vi "Drive Controller.vi"(8 "error in":errorcluster) -> ()   [LabVIEW 2019]
doc: "This VI executes continuously carrying out the current operation and responding to updates or new operation requests. It will often contain the timing or control code that is difficult to place directly in TeleOp. This VI generally opens all sensors and motors and isolates the rest of the robot code from knowing implementation details of how the operations are carried out."
uses:
  <vilib>/Rock Robotics/WPI/Framework/Completion Status.ctl
  Drive Setpoints.ctl
  Drive Operations.ctl
  <vilib>/Rock Robotics/WPI/ThirdParty/REV Robotics/SPARK MAX/Typedef/Spark MAX Control Type.ctl
  Odometry/ADIS16470/Typedef/ADIS16470 Hardware Configuration.ctl
  <vilib>/Rock Robotics/WPI/SPI/WPI_SPIMode.ctl
  <vilib>/Rock Robotics/SystemInterfaces/DIO/FPGA_DIOChannel.ctl
  <vilib>/Rock Robotics/SystemInterfaces/spilib/spi_bus.ctl
  <vilib>/Rock Robotics/WPI/ThirdParty/WPILib Extensions/Geometry/Typedef/Pose2d.ctl
  <vilib>/Rock Robotics/WPI/ThirdParty/WPILib Extensions/Geometry/Typedef/Translation2d.ctl
  <vilib>/Rock Robotics/WPI/ThirdParty/WPILib Extensions/Geometry/Typedef/Rotation2d.ctl
  <vilib>/Rock Robotics/WPI/Gyro/WPI_GyroDevRef.ctl
  <vilib>/Rock Robotics/SystemInterfaces/AI/FPGA_AIChannel.ctl
  CAN Functions/SPARKMAX6Motor.ctl
  <vilib>/Rock Robotics/WPI/MotorControl/WPI_MotorControlDeviceRef.ctl
  <vilib>/Rock Robotics/WPI/MotorControl/WPI_MotorControlType.ctl
  <vilib>/Rock Robotics/SystemInterfaces/DIO/FPGA_DIOPWMChannel.ctl
  <vilib>/Rock Robotics/WPI/PWM/WPI_PWMDeadband.ctl
  <vilib>/Rock Robotics/WPI/ThirdParty/WPILib Extensions/Controller/PID/Typedef/PID Controller State.ctl
  Odometry/ADIS16470/Typedef/ADIS16470 Calibration Time.ctl
  Odometry/Typedef/Odometry.ctl
  Odometry/Typedef/Velocity Data.ctl
  Pure Pursuit/Typedef/Pure Pursuit Telemetry.ctl
  Pure Pursuit/Typedef/Path Point.ctl
  <vilib>/Rock Robotics/WPI/ThirdParty/WPILib Extensions/Trajectory/Typedef/Trajectory State.ctl
  <vilib>/Rock Robotics/WPI/Counter/WPI_CounterDigitalInputToDigitalSource.vi
  Odometry/Odometry Set.vi
  <vilib>/ptbypt/NI_PtbyPt.lvlib
  Pure Pursuit/Pure Pursuit.lvlib
panel:
  in  "Drive Distance Tolerance":dbl format="%#_13g"
  in  "ADIS16470 Config":T1={"SPI Clock Rate (Hz)"=2000000.0, "IMU SPI Mode (3)"=enum."Mode 3 (Clk Idle High,Sample on Trailing)", "IMU Reset Pin"=enum."SPI Port CS2", "IMU SPI Bus"=enum."SPI On-Board, CS0", "IMU Data Ready Pin"=enum."SPI Port CS1", "Stall Config"={"Pow2BytesPerRead"=1, "StallTicks"=1000, "CsToSclkTicks"=5}}
  in  "Trackwidth":dbl=0.6716296994500001
  in  "Control Mode":T5
  in  "Tab Control":T6(tab)=enum."Settings"
  in  "Interactive Values":T7
  in  "Buttons":cluster{"Execute Cmd":bool, "Abort Cmd":bool}
  out "Command Timing":cluster{"Start Time (ms)":u32, "Iterations":i32}={"Start Time (ms)"=2524017, "Iterations"=0}
  out "Status":T9
  in  "PID Constants Drivetrain":T10={"P Gain"=1.0, "I Gain"=0.0, "D Gain"=0.0, "F Gain"=0.0, "I Zone"=0.0, "Min Output"=-1.0, "Max Output"=1.0} {"Max Output" min=-1.0 max=1.0 step=0.01; "Min Output" min=-1.0 max=1.0 step=0.01; "I Zone" step=0.01; "F Gain" step=0.01; "D Gain" step=0.01; "I Gain" step=0.01; "P Gain" min=0.0 step=0.01}
  in  "Trackwidth":dbl=0.6716296994500001 format="%#_13g"
  in  "Max Velocity":dbl=2.0
  in  "Max Accel":dbl=4.0
  in  "Lookahead":dbl=18.0
  in  "kffv":dbl
  in  "kffa":dbl=0.05
  in  "Feed Forward":cluster{"kS":dbl, "kV":dbl, "kA":dbl}={"kS"=0.162, "kV"=2.71, "kA"=0.468}
  in  "Encoder Factor":dbl=0.00030795
  out "Pose":T11
  in  "Value":dbl
  in  "Run":bool
  out "Waveform Chart":dbl(graph)
  out "XY Graph":cluster{"X":dbl, "Y":dbl}[](graph)
  in  "Test":string(combo)="quasi-static ramp"
  out "Telemetry":cluster{dbl[], dbl[]}[](graph)
  in  "Output Range":cluster{"output high":dbl, "output low":dbl}
  in  "Profiled Contraints":T14
  in  "PIDF Gains":cluster{"Kp":dbl, "Ki":dbl, "Kd":dbl, "Kf":dbl}
  in  "Gyro PIDF":cluster{"Kp":dbl, "Ki":dbl, "Kd":dbl, "Kf":dbl}={"Kp"=0.05, "Ki"=0.0, "Kd"=0.0, "Kf"=0.0} {"Kf" format="%.3f"; "Kd" format="%.3f"; "Ki" format="%.3f"; "Kp" format="%.3f"}
  out "Current\nCmd":string="Started at  20:49:40.426\nDefault: Reserve,  L 0.0, R 0.0, D 0.000000"
  # "Click here to set min"
  # "Interactive Command: You may fill in the settings for a command\nand schedule it with the Execute button. You can observe and abort\nany command while fine tuning the code for the controller."
  # "Pure Pursuit"
  # "Velocity Control is the Output (m/s)"
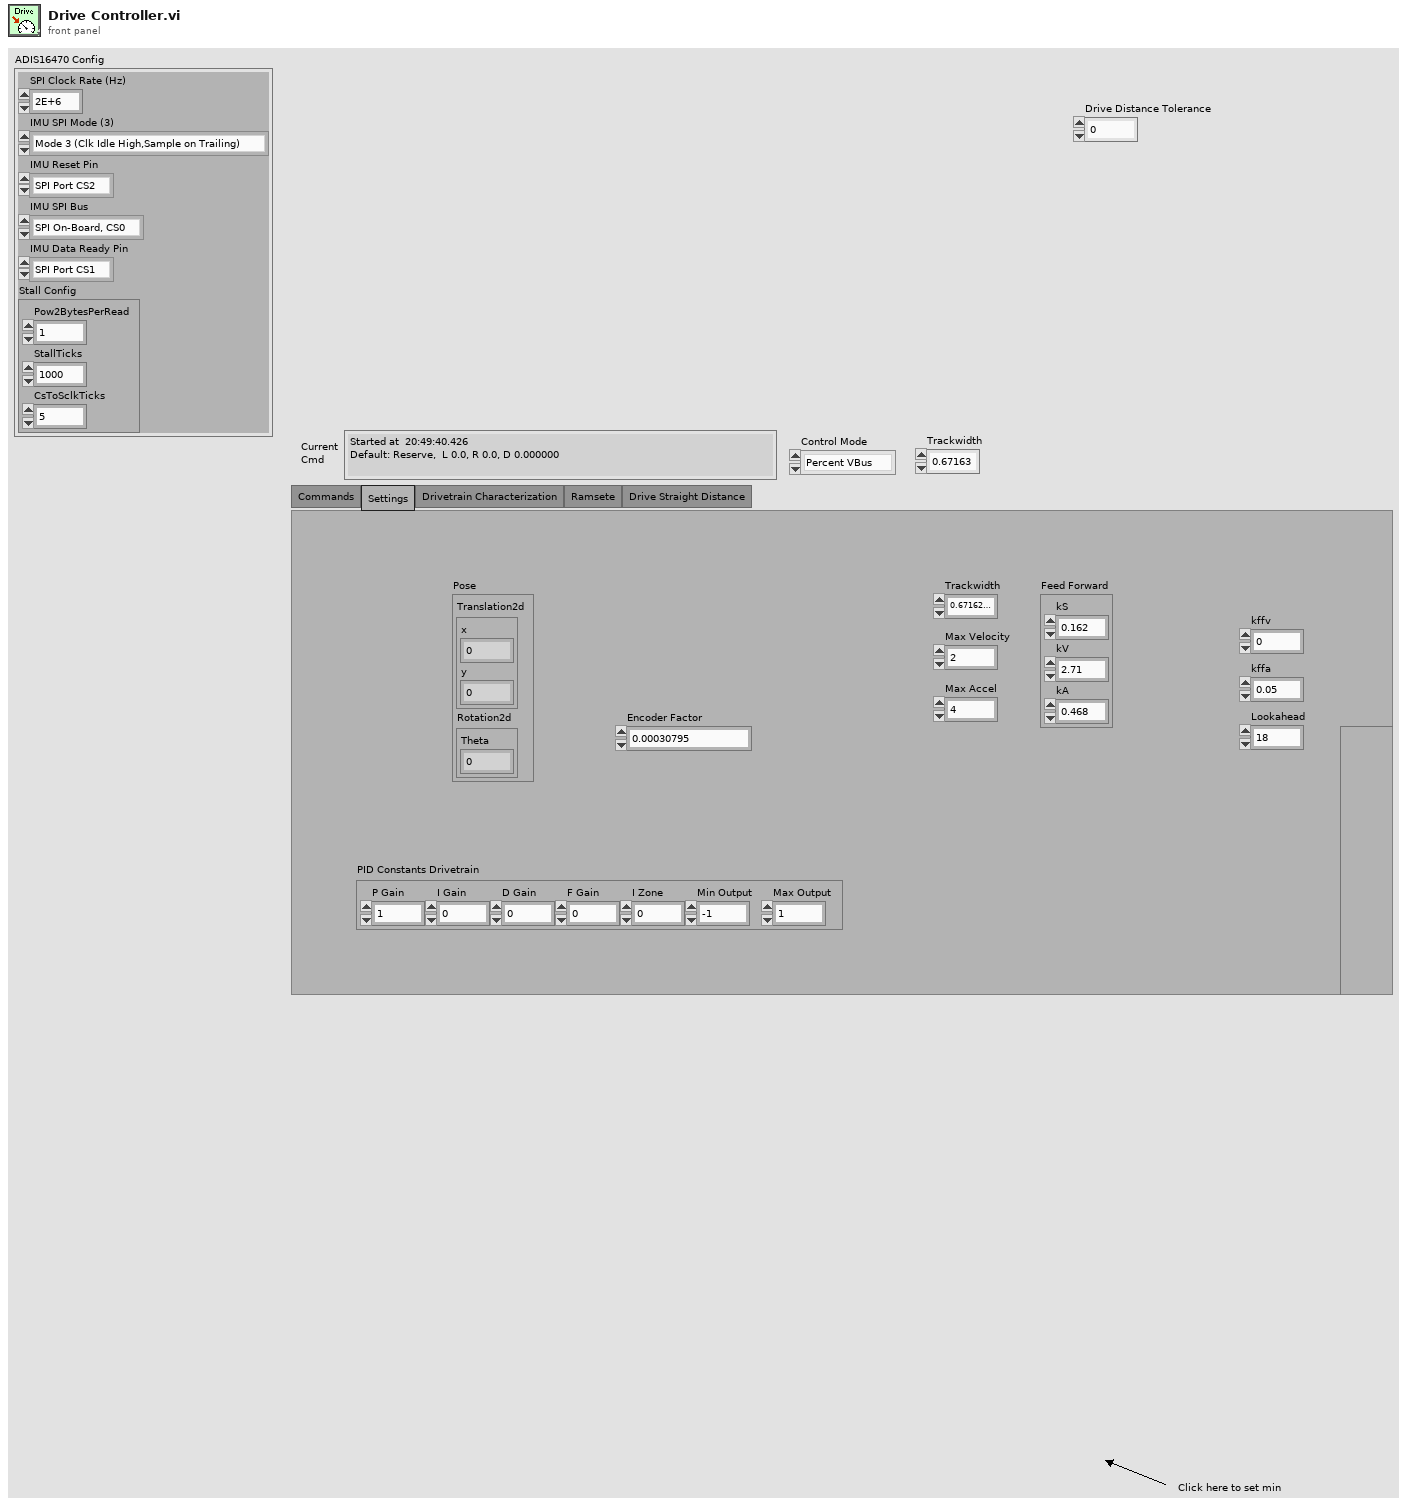
[diagram p1: front panel]
types:
  T1 = typedef "ADIS16470 Hardware Configuration.ctl" = cluster{"SPI Clock Rate (Hz)":dbl, "IMU SPI Mode (3)":T2, "IMU Reset Pin":T3, "IMU SPI Bus":T4, "IMU Data Ready Pin":T3, "Stall Config":cluster{"Pow2BytesPerRead":u8, "StallTicks":u16, "CsToSclkTicks":u8}}
  T2 = typedef "WPI_SPIMode.ctl" = enum16{"Mode 0 (Clk Idle Low,Sample on Leading)", "Mode 1 (Clk Idle Low,Sample on Trailing)", "Mode 2 (Clk Idle High,Sample on Leading)", "Mode 3 (Clk Idle High,Sample on Trailing)"}
  T3 = typedef "FPGA_DIOChannel.ctl" = enum8{"DIO 0", "DIO 1", "DIO 2", "DIO 3", "DIO 4", "DIO 5", "DIO 6", "DIO 7", "DIO 8", "DIO 9", "DIO MXP 0", "DIO MXP 1", "DIO MXP 2", "DIO MXP 3", "DIO MXP 4", "DIO MXP 5", "DIO MXP 6", "DIO MXP 7", "DIO MXP 8", "DIO MXP 9", "DIO MXP 10", "DIO MXP 11", "DIO MXP 12", "DIO MXP 13", "DIO MXP 14", "DIO MXP 15", "SPI Port CS1", "SPI Port CS2", "SPI Port CS3", "SPI Port MISO", "SPI Port MOSI", "Invalid"}
  T4 = typedef "spi_bus.ctl" = enum16{"SPI On-Board, CS0", "SPI On-Board, CS1", "SPI On-Board, CS2", "SPI On-Board, CS3", "SPI MXP", "Invalid"}
  T5 = typedef "Spark MAX Control Type.ctl" = enum16{"Percent VBus", "Voltage", "Velocity", "Position", "Smart Motion", "Current", "Smart Velocity"}
  T6 = enum32{"Commands", "Settings", "Drivetrain Characterization", "Ramsete", "Drive Straight Distance"}
  T7 = typedef "Drive Setpoints.ctl" = cluster{"Operation":T8, "Left Setpoint":dbl, "Right Setpoint":dbl, "Duration":dbl, "Data":variant}
  T8 = typedef "Drive Operations.ctl" = enum16{"Reserve", "Read Current", "Immediate", "Drive for Time", "Drive for Distance", "Turn to Angle", "Drivetrain Char", "Pure Pursuit", "Ramsete"}
  T9 = typedef "Completion Status.ctl" = enum16{"Successful", "Aborted", "Incomplete"}
  T10 = cluster{"P Gain":dbl, "I Gain":dbl, "D Gain":dbl, "F Gain":dbl, "I Zone":dbl, "Min Output":dbl, "Max Output":dbl}
  T11 = typedef "Pose2d.ctl" = cluster{"Translation2d":T12, "Rotation2d":T13}
  T12 = typedef "Translation2d.ctl" = cluster{"x":dbl, "y":dbl}
  T13 = typedef "Rotation2d.ctl" = cluster{"Theta":dbl}
  T14 = cluster{"Max Velocity":dbl, "Max Acceleration":dbl}
  T15 = typedef "WPI_GyroDevRef.ctl" = cluster{"DevStatus":errorcluster, "Analog Channel":T16, "Gain (VoltsPerDegree/Second)":dbl, "Gyro Type":enum16{"Analog", "XRS450"}, "Handle":i32, "SPI Bus":T4, "Device Found":bool, "Sample Rate":dbl, "Calibrate On Open":bool, "Offset":dbl}
  T16 = typedef "FPGA_AIChannel.ctl" = enum8{"AI 0", "AI 1", "AI 2", "AI 3", "AI MXP 0", "AI MXP 1", "AI MXP 2", "AI MXP 3", "Invalid"}
  T17 = typedef "SPARKMAX6Motor.ctl" = cluster{"FrontLeftMaster":T18, "FrontLeftSlave1":T18, "FrontLeftSlave2":T18, "FrontRightMaster":T18, "FrontRightSlave1":T18, "FrontRightSlave2":T18}
  T18 = typedef "WPI_MotorControlDeviceRef.ctl" = cluster{"DeviceStatus":errorcluster, "Type":T19, "PWM":cluster{"PWM Channel":T20, "DeadBand":T21}, "CAN":cluster{"Device Number":u8, "SetOutput VI Ref":variant, "GetOutput VI Ref":variant, "Enable VI Ref":variant, "Disable VI Ref":variant, "Data":variant}, "Invert":bool, "DIO PWM":cluster{"PWM \"Enable\" Channel":T20, "DIOChannel":T3, "PWM Rate":dbl}}
  T19 = typedef "WPI_MotorControlType.ctl" = enum16{"PWM", "CAN", "DIO PWM"}
  T20 = typedef "FPGA_DIOPWMChannel.ctl" = enum8{"PWM 0", "PWM 1", "PWM 2", "PWM 3", "PWM 4", "PWM 5", "PWM 6", "PWM 7", "PWM 8", "PWM 9", "PWM MXP 0", "PWM MXP 1", "PWM MXP 2", "PWM MXP 3", "PWM MXP 4", "PWM MXP 5", "PWM MXP 6", "PWM MXP 7", "PWM MXP 8", "PWM MXP 9", "Invalid"}
  T21 = typedef "WPI_PWMDeadband.ctl" = cluster{"Name":string, "maxPositivePwm":i32, "minPositivePwm":i32, "centerPwm":i32, "maxNegativePwm":i32, "minNegativePwm":i32, "angularRange":u16}
  T22 = cluster{"Gyro":T15, "Drivetrain":T17, "PID Ref":refnum<data-value>}
  T23 = typedef "ADIS16470 Calibration Time.ctl" = enum16{"32ms", "64ms", "128ms", "256ms", "512ms", "1s", "2s", "4s", "8s", "16s", "32s", "64s"}
  T24 = typedef "WPI_DigitalInputDevRef.ctl" = cluster{"DevStatus":errorcluster, "DIO Channel":T3}
  T25 = typedef "FPGA_CounterEncoderSourceConvertionLVSourceType.ctl" = cluster{"DevStatus":errorcluster, "AnalogTriggerMode?":bool, "DigitalMode":cluster{"DIO Channel":T26}, "AnalogTriggerMode":cluster{"AnalogTriggerIndex":T27, "OutputType":T28}}
  T26 = typedef "FPGA_DIODigitalSourceChannel.ctl" = enum8{"DIO 0", "DIO 1", "DIO 2", "DIO 3", "DIO 4", "DIO 5", "DIO 6", "DIO 7", "DIO 8", "DIO 9", "DIO MXP 0", "DIO MXP 1", "DIO MXP 2", "DIO MXP 3", "DIO MXP 4", "DIO MXP 5", "DIO MXP 6", "DIO MXP 7", "DIO MXP 8", "DIO MXP 9", "DIO MXP 10", "DIO MXP 11", "DIO MXP 12", "DIO MXP 13", "DIO MXP 14", "DIO MXP 15", "SPI Port CS1", "SPI Port CS2", "SPI Port CS3", "SPI Port MISO", "SPI Port MOSI", "Disabled"}
  T27 = typedef "FPGA_AnalogTriggerIndex.ctl" = enum8{"Trig 0", "Trig 1", "Trig 2", "Trig 3", "Trig 4", "Trig 5", "Trig 6", "Trig 7", "Invalid"}
  T28 = typedef "FPGA_AnalogTriggerOutType.ctl" = enum16{"InWindow", "TriggerState", "Rising", "Falling"}
  T29 = typedef "WPI_EncoderDevRef.ctl" = cluster{"DevStatus":errorcluster, "EncoderIndex":T30, "CounterIndex":T31, "DistancePerCount":dbl, "Decoding Type":T32}
  T30 = typedef "FPGA_EncoderIdx.ctl" = enum8{"Enc 0", "Enc 1", "Enc 2", "Enc 3", "Enc 4", "Enc 5", "Enc 6", "Enc 7", "Invalid"}
  T31 = typedef "FPGA_CounterCtrSystemIndex.ctl" = enum8{"Ctr 0", "Ctr 1", "Ctr 2", "Ctr 3", "Ctr 4", "Ctr 5", "Ctr 6", "Ctr 7", "Invalid"}
  T32 = typedef "WPI_EncoderType.ctl" = enum16{"1x", "2x", "4x"}
  T33 = typedef "ADIS16470 Device Reference.ctl" = cluster{"DevStatus":errorcluster, "Hardware Config":T1, "Calibration Complete":refnum<notifier>, "Status FIFO":refnum<k33>, "Last Value Reference":refnum<data-value>, "Sychronous Process VI":T34, "Cmd FIFO":refnum<k33>, "Source":T25, "Data FIFO":refnum<k33>, "Calibration Time":T23}
  T34 = typedef "ADIS16470 Process.ctl" = refnum<vi>
  T35 = typedef "Command Status Info.ctl" = cluster{"Name":string, "Status":T9, "notifier out":T36}
  T36 = typedef "Completion Notifier.ctl" = refnum<notifier>
  T37 = cluster{"SubSystem Data":T7, cluster{"Start Time (ms)":u32, "Iterations":i32}, cluster{"Command Info":T35, "Description":string, "Default Command":T7, "queue out":refnum<queue>, "Subsystem Name":string}}
  T38 = typedef "Pure Pursuit.lvlib/Pure Pursuit Telemetry.ctl" = cluster{"Target Point":T39, "Close Point":T39, "Curvature":dbl, "index out":i32}
  T39 = typedef "Pure Pursuit.lvlib/Path Point.ctl" = cluster{"x":dbl, "y":dbl, "heading":dbl, "curvature":dbl, "total distance":dbl, "velocity expected":dbl}
  T40 = typedef "Trajectory State.ctl" = cluster{"t":dbl, "velocity":dbl, "acceleration":dbl, "pose":T11, "curvature":dbl}
  T41 = typedef "Odometry.ctl" = cluster{"Left Encoder":dbl, "Right Encoder":dbl, "Late Iterations":u32, "Pose2d":T11}
  T42 = typedef "Velocity Data.ctl" = cluster{"Right Velocity Raw":sgl, "Left Velocity Raw":sgl, "Left Setpoint":dbl, "Right Setpoint":dbl}
  T43 = cluster{"SubSystem Data":T7, cluster{"Start Time (ms)":u32, "Iterations":i32}, "Default Command Arguments":cluster{"Command Info":T35, "Description":string, "Default Command":T7, "queue out":refnum<queue>, "Subsystem Name":string}}
  T44 = cluster{"P Gain":bool, "I Gain":bool, "D Gain":bool, "F Gain":bool, "I Zone":bool, "Min Output":bool, "Max Output":bool}
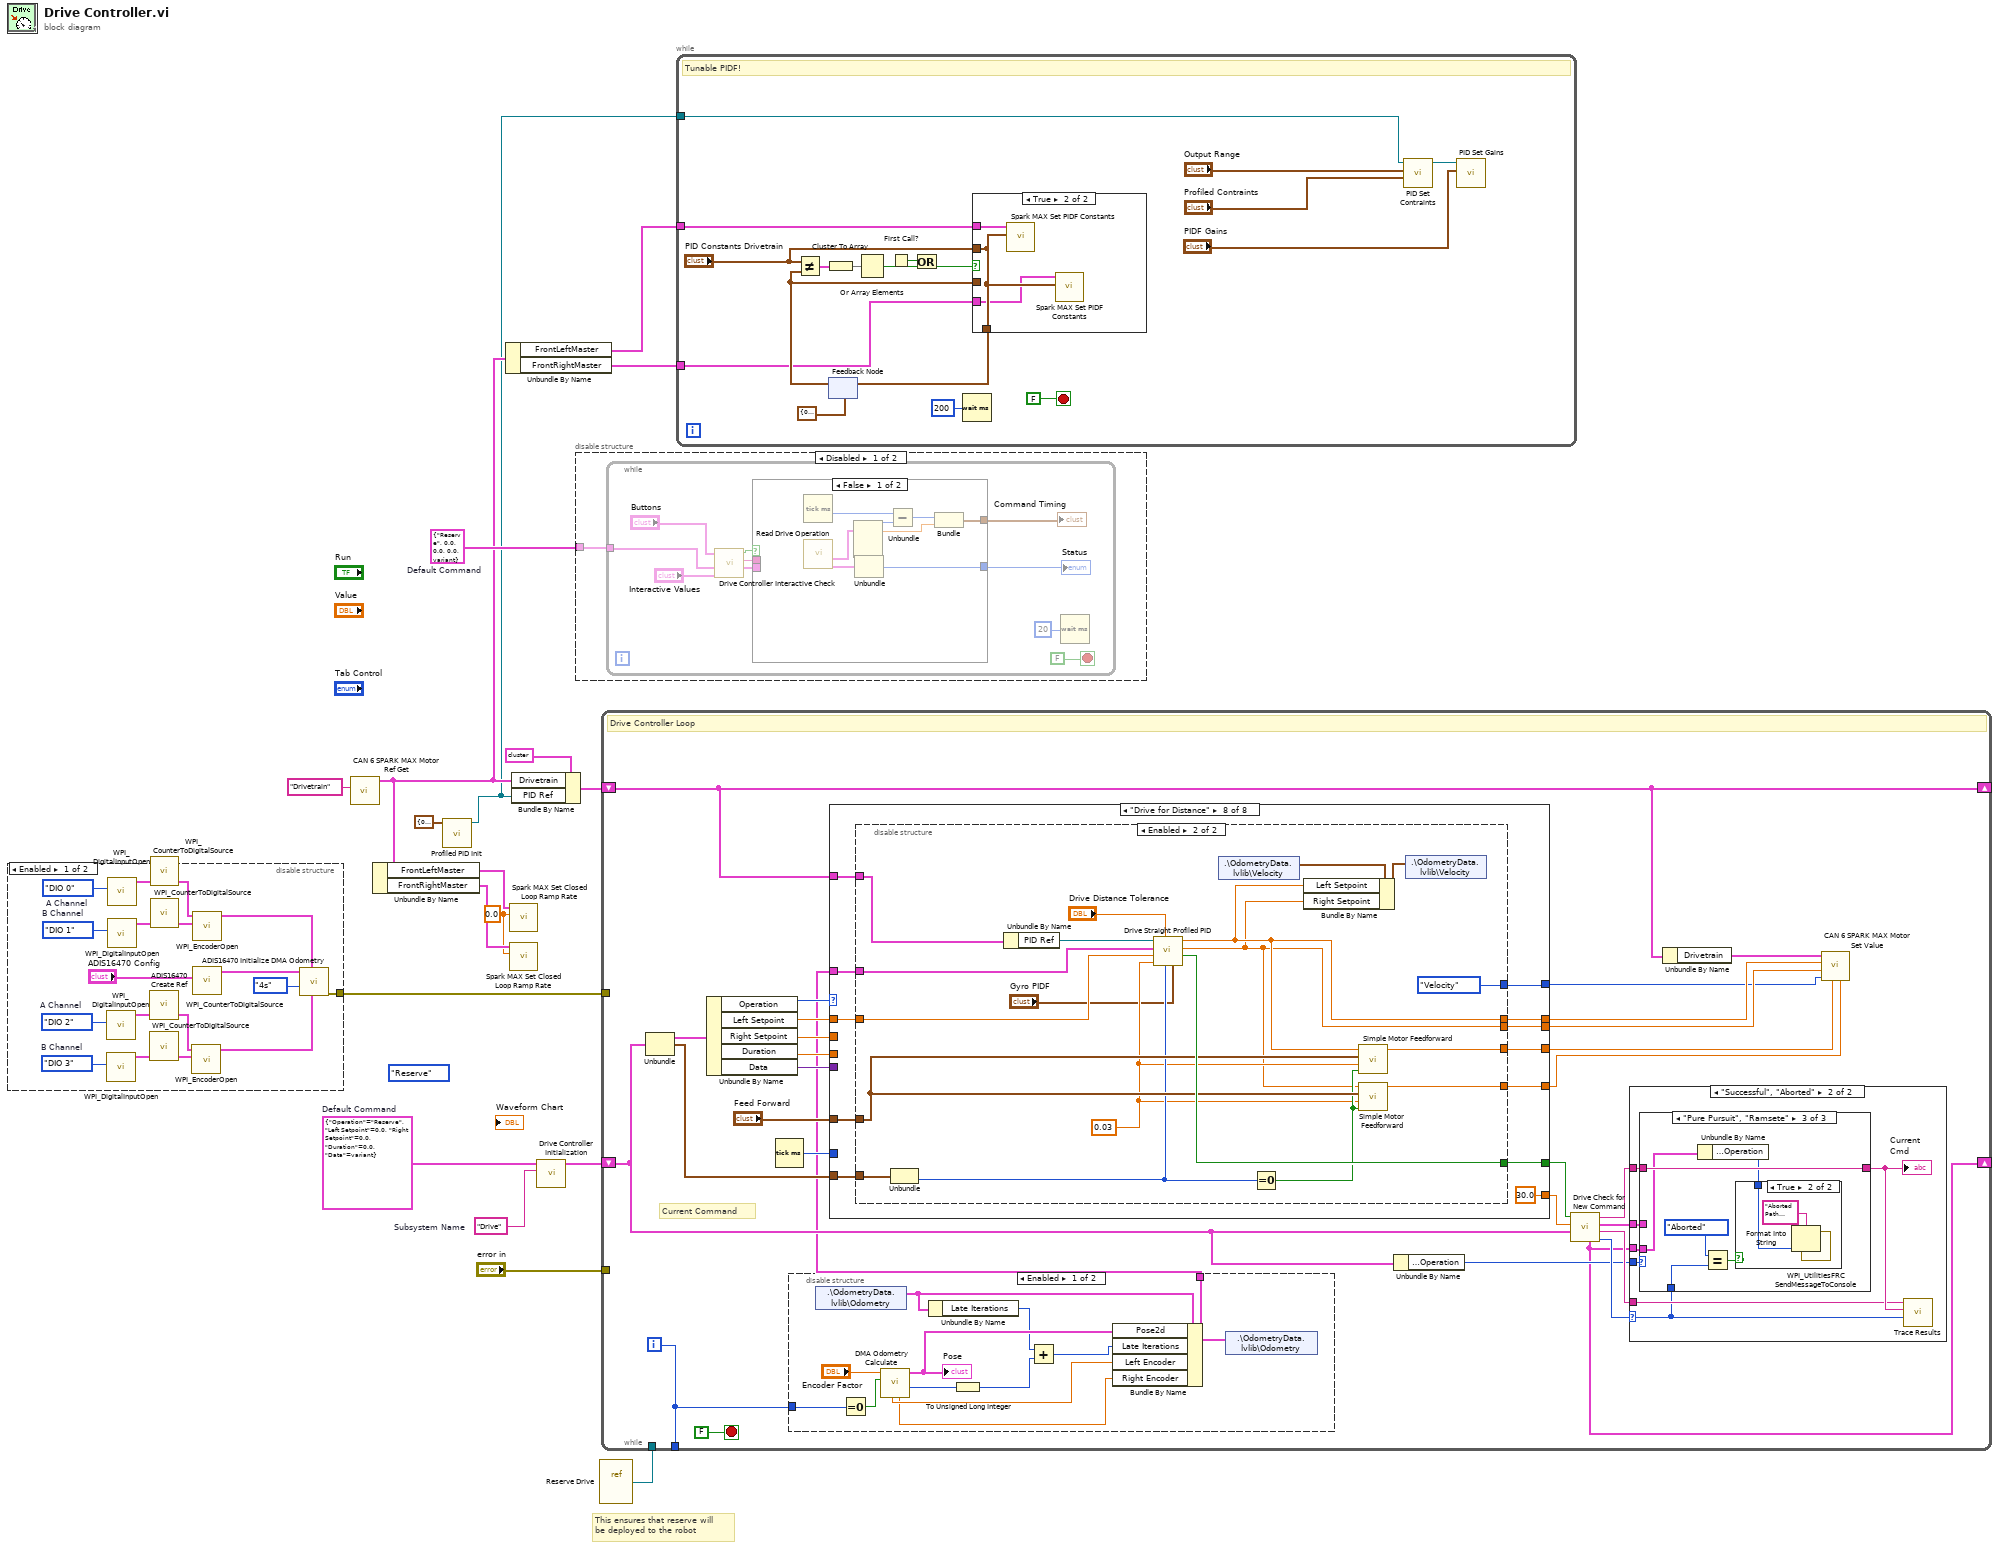
[diagram p0: block diagram]
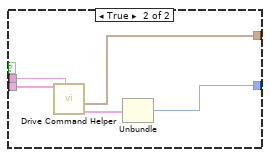
[diagram p3: hidden frame]
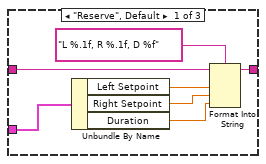
[diagram p7: hidden frame]
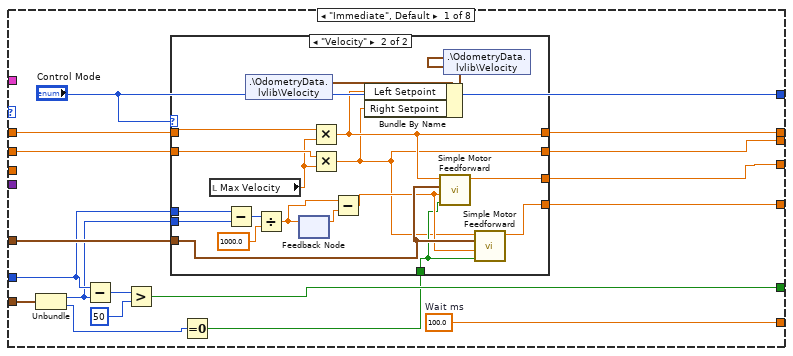
[diagram p10: hidden frame]
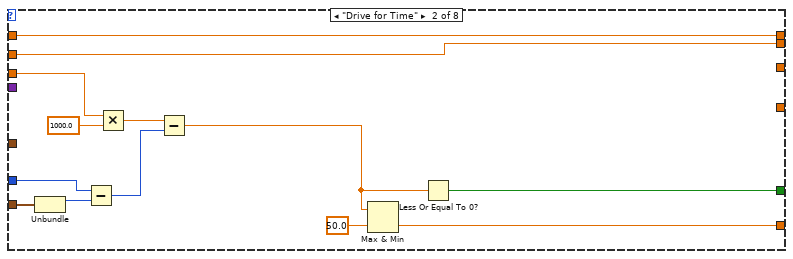
[diagram p12: hidden frame]
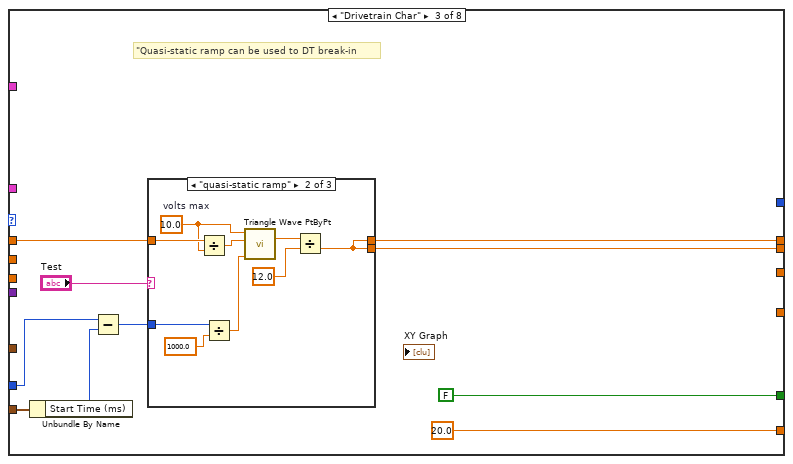
[diagram p13: hidden frame]
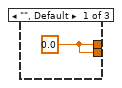
[diagram p14: hidden frame]
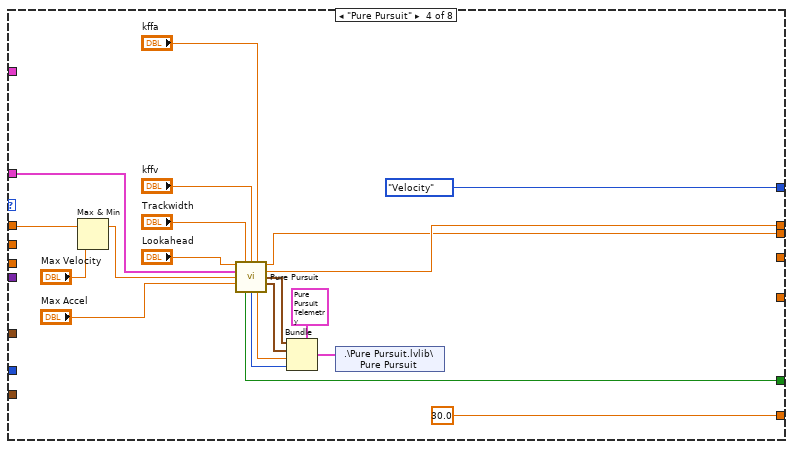
[diagram p16: hidden frame]
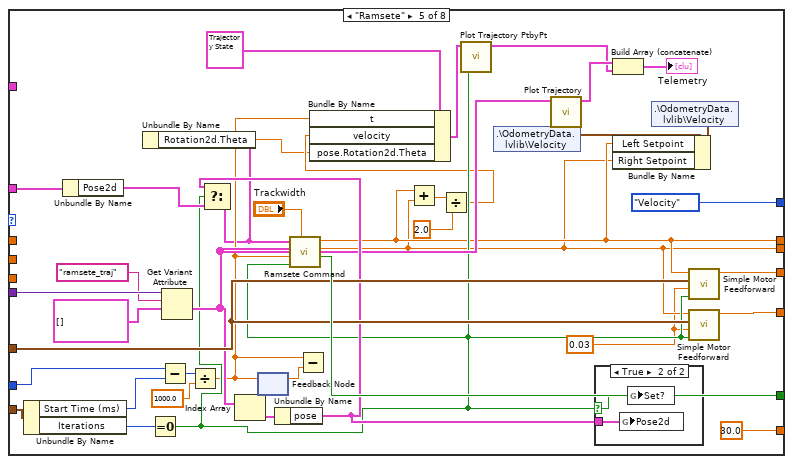
[diagram p17: hidden frame]
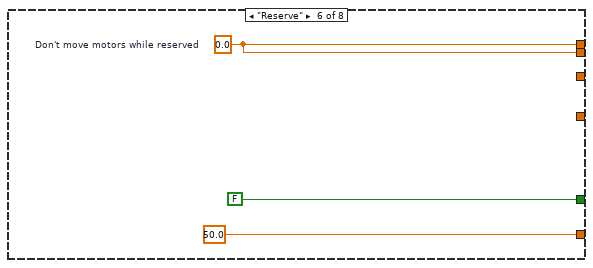
[diagram p19: hidden frame]
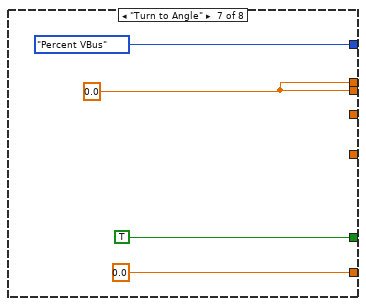
[diagram p20: hidden frame]
diagram:
  w3 = sgl 0.0 ("Seconds from neutral to full (0)")
  (unwired) Drive_Operations."Reserve" ("Operation")
  w13 = T7 {"Operation"=enum."Reserve", "Left Setpoint"=0.0, "Right Setpoint"=0.0, "Duration"=0.0, "Data"=variant}  # Default Command
  w14 = T7 {"Operation"=enum."Reserve", "Left Setpoint"=0.0, "Right Setpoint"=0.0, "Duration"=0.0, "Data"=variant}  # Default Command
  w18 = "Drive"  # Subsystem Name
  # "This ensures that reserve will\nbe deployed to the robot"
  n1 = disable-structure shown="Enabled" {
    disable-tunnel: [w36 _] -> w7
    frame Enabled {
      w23 = FPGA_DIOChannel."DIO 1"  # B Channel
      w24 = FPGA_DIOChannel."DIO 0"  # A Channel
      w34 = FPGA_DIOChannel."DIO 3"  # B Channel
      w33 = FPGA_DIOChannel."DIO 2"  # A Channel
      n2 = call <vilib>:"WPI_DigitalInputOpen.vi"("DIO Channel"=w33) -> ("DigitalInputDevRef"=w30:T24)  [unwired: 1 in, 9 out]
      n3 = call <vilib>:"WPI_DigitalInputOpen.vi"("DIO Channel"=w34) -> ("DigitalInputDevRef"=w31:T24)  [unwired: 1 in, 9 out]
      n4 = call <vilib>:"WPI_DigitalInputOpen.vi"("DIO Channel"=w24) -> ("DigitalInputDevRef"=w27:T24)  [unwired: 1 in, 9 out]
      n5 = call <vilib>:"WPI_DigitalInputOpen.vi"("DIO Channel"=w23) -> ("DigitalInputDevRef"=w26:T24)  [unwired: 1 in, 9 out]
      n6 = call-poly <vilib>:"WPI_CounterToDigitalSource.vi"("DigitalInputDevRef"=w30) -> ("Digital Source"=w29:T25)  [unwired: 6 out]
      n7 = call-poly <vilib>:"WPI_CounterToDigitalSource.vi"("DigitalInputDevRef"=w31) -> ("Digital Source"=w32:T25)  [unwired: 6 out]
      n8 = call-poly <vilib>:"WPI_CounterToDigitalSource.vi"("DigitalInputDevRef"=w27) -> ("Digital Source"=w28:T25)  [unwired: 6 out]
      n9 = call-poly <vilib>:"WPI_CounterToDigitalSource.vi"("DigitalInputDevRef"=w26) -> ("Digital Source"=w25:T25)  [unwired: 6 out]
      n10 = call <vilib>:"WPI_EncoderOpen.vi"("BSource"=w32, "ASource"=w29) -> ("EncoderDevRef"=w20:T29)  [unwired: 6 in, 3 out]
      n11 = call <vilib>:"WPI_EncoderOpen.vi"("BSource"=w25, "ASource"=w28) -> ("EncoderDevRef"=w21:T29)  [unwired: 6 in, 3 out]
      n12 = call "ADIS16470 Create Ref.vi"("Hardware Config"="ADIS16470 Config") -> ("ADIS16470DevRef"=w22:T33)  [unwired: 9 in, 1 out]
      n13 = call "ADIS16470 Initialize DMA Odometry.vi"("Encoder R"=w20, "Encoder L"=w21, "Calibration Time"=ADIS16470_Calibration_Time."4s", "ADIS16470DevRef"=w22) -> ("error out"=w36:errorcluster)  [unwired: 7 in]
    }
    frame Disabled {
    }
  }
  n14 = call "CAN 6 SPARK MAX Motor Ref Get.vi"("refnum name"="Drivetrain") -> ("TalonSRX6MotorRef out"=w6:T17)  [unwired: 9 in, 1 out]
  n15 = Unbundle By Name(w6) -> ("FrontLeftMaster"=w5:T18, "FrontRightMaster"=w4:T18)
  n16 = call <vilib>:"Profiled PID Init.vi"("PIDF Gains"=cluster{"Kp":dbl, "Ki":dbl, "Kd":dbl, "Kf":dbl} {"Kp"=0.0, "Ki"=0.0, "Kd"=0.0, "Kf"=0.0}) -> ("PID Ref"=w1:refnum<data-value>)  [unwired: 10 in]
  n17 = Unbundle By Name(w6) -> ("FrontLeftMaster"=w9:T18, "FrontRightMaster"=w8:T18)
  n18 = call <vilib>:"Spark MAX Set Closed Loop Ramp Rate.vi"("Seconds from neutral to full (0)"=w3, "MotorControlDeviceRef in"=w5) -> ()  [unwired: 8 in, 2 out]
  n19 = call <vilib>:"Spark MAX Set Closed Loop Ramp Rate.vi"("Seconds from neutral to full (0)"=w3, "MotorControlDeviceRef in"=w4) -> ()  [unwired: 8 in, 2 out]
  n20 = Bundle By Name(cluster=T22 {"Gyro"={"DevStatus"={"status"=FALSE, "code"=0, "source"=""}, "Analog Channel"=enum."Invalid", "Gain (VoltsPerDegree/Second)"=0.0, "Gyro Type"=enum."Analog", "Handle"=0, "SPI Bus"=enum."Invalid", "Device Found"=FALSE, "Sample Rate"=1.0, "Calibrate On Open"=FALSE, "Offset"=0.0}, "Drivetrain"={"FrontLeftMaster"={"DeviceStatus"={"status"=FALSE, "code"=0, "source"=""}, "Type"=enum."PWM", "PWM"={"PWM Channel"=enum."PWM 1", "DeadBand"={"Name"="", "maxPositivePwm"=0, "minPositivePwm"=0, "centerPwm"=0, "maxNegativePwm"=0, "minNegativePwm"=0, "angularRange"=0}}, "CAN"={"Device Number"=0, "SetOutput VI Ref"=variant(enum8{"Percent VBus", "Current", "Speed", "Position", "Voltage"} enum."Percent VBus"), "GetOutput VI Ref"=variant(refnum<k1> refnum), "Enable VI Ref"=variant(dbl 12.0), "Disable VI Ref"=variant(enum8{"Percent VBus", "Speed", "Position", "Slave", "Unchanged / Invalid", "Voltage Compensation", "Current", "Motion Profile"} enum."Percent VBus"), "Data"=variant}, "Invert"=FALSE, "DIO PWM"={"PWM \"Enable\" Channel"=enum."Invalid", "DIOChannel"=enum."Invalid", "PWM Rate"=0.0}}, "FrontLeftSlave1"={"DeviceStatus"={"status"=FALSE, "code"=0, "source"=""}, "Type"=enum."PWM", "PWM"={"PWM Channel"=enum."PWM 1", "DeadBand"={"Name"="", "maxPositivePwm"=0, "minPositivePwm"=0, "centerPwm"=0, "maxNegativePwm"=0, "minNegativePwm"=0, "angularRange"=0}}, "CAN"={"Device Number"=0, "SetOutput VI Ref"=variant(enum8{"Percent VBus", "Current", "Speed", "Position", "Voltage"} enum."Percent VBus"), "GetOutput VI Ref"=variant(refnum<k1> refnum), "Enable VI Ref"=variant(dbl 12.0), "Disable VI Ref"=variant(enum8{"Percent VBus", "Speed", "Position", "Slave", "Unchanged / Invalid", "Voltage Compensation", "Current", "Motion Profile"} enum."Percent VBus"), "Data"=variant}, "Invert"=FALSE, "DIO PWM"={"PWM \"Enable\" Channel"=enum."Invalid", "DIOChannel"=enum."Invalid", "PWM Rate"=0.0}}, "FrontLeftSlave2"={"DeviceStatus"={"status"=FALSE, "code"=0, "source"=""}, "Type"=enum."PWM", "PWM"={"PWM Channel"=enum."PWM 1", "DeadBand"={"Name"="", "maxPositivePwm"=0, "minPositivePwm"=0, "centerPwm"=0, "maxNegativePwm"=0, "minNegativePwm"=0, "angularRange"=0}}, "CAN"={"Device Number"=0, "SetOutput VI Ref"=variant(enum8{"Percent VBus", "Current", "Speed", "Position", "Voltage"} enum."Percent VBus"), "GetOutput VI Ref"=variant(refnum<k1> refnum), "Enable VI Ref"=variant(dbl 12.0), "Disable VI Ref"=variant(enum8{"Percent VBus", "Speed", "Position", "Slave", "Unchanged / Invalid", "Voltage Compensation", "Current", "Motion Profile"} enum."Percent VBus"), "Data"=variant}, "Invert"=FALSE, "DIO PWM"={"PWM \"Enable\" Channel"=enum."Invalid", "DIOChannel"=enum."Invalid", "PWM Rate"=0.0}}, "FrontRightMaster"={"DeviceStatus"={"status"=FALSE, "code"=0, "source"=""}, "Type"=enum."PWM", "PWM"={"PWM Channel"=enum."PWM 1", "DeadBand"={"Name"="", "maxPositivePwm"=0, "minPositivePwm"=0, "centerPwm"=0, "maxNegativePwm"=0, "minNegativePwm"=0, "angularRange"=0}}, "CAN"={"Device Number"=0, "SetOutput VI Ref"=variant(enum8{"Percent VBus", "Current", "Speed", "Position", "Voltage"} enum."Percent VBus"), "GetOutput VI Ref"=variant(refnum<k1> refnum), "Enable VI Ref"=variant(dbl 12.0), "Disable VI Ref"=variant(enum8{"Percent VBus", "Speed", "Position", "Slave", "Unchanged / Invalid", "Voltage Compensation", "Current", "Motion Profile"} enum."Percent VBus"), "Data"=variant}, "Invert"=FALSE, "DIO PWM"={"PWM \"Enable\" Channel"=enum."Invalid", "DIOChannel"=enum."Invalid", "PWM Rate"=0.0}}, "FrontRightSlave1"={"DeviceStatus"={"status"=FALSE, "code"=0, "source"=""}, "Type"=enum."PWM", "PWM"={"PWM Channel"=enum."PWM 1", "DeadBand"={"Name"="", "maxPositivePwm"=0, "minPositivePwm"=0, "centerPwm"=0, "maxNegativePwm"=0, "minNegativePwm"=0, "angularRange"=0}}, "CAN"={"Device Number"=0, "SetOutput VI Ref"=variant(enum8{"Percent VBus", "Current", "Speed", "Position", "Voltage"} enum."Percent VBus"), "GetOutput VI Ref"=variant(refnum<k1> refnum), "Enable VI Ref"=variant(dbl 12.0), "Disable VI Ref"=variant(enum8{"Percent VBus", "Speed", "Position", "Slave", "Unchanged / Invalid", "Voltage Compensation", "Current", "Motion Profile"} enum."Percent VBus"), "Data"=variant}, "Invert"=FALSE, "DIO PWM"={"PWM \"Enable\" Channel"=enum."Invalid", "DIOChannel"=enum."Invalid", "PWM Rate"=0.0}}, "FrontRightSlave2"={"DeviceStatus"={"status"=FALSE, "code"=0, "source"=""}, "Type"=enum."PWM", "PWM"={"PWM Channel"=enum."PWM 1", "DeadBand"={"Name"="", "maxPositivePwm"=0, "minPositivePwm"=0, "centerPwm"=0, "maxNegativePwm"=0, "minNegativePwm"=0, "angularRange"=0}}, "CAN"={"Device Number"=0, "SetOutput VI Ref"=variant(enum8{"Percent VBus", "Current", "Speed", "Position", "Voltage"} enum."Percent VBus"), "GetOutput VI Ref"=variant(refnum<k1> refnum), "Enable VI Ref"=variant(dbl 12.0), "Disable VI Ref"=variant(enum8{"Percent VBus", "Speed", "Position", "Slave", "Unchanged / Invalid", "Voltage Compensation", "Current", "Motion Profile"} enum."Percent VBus"), "Data"=variant}, "Invert"=FALSE, "DIO PWM"={"PWM \"Enable\" Channel"=enum."Invalid", "DIOChannel"=enum."Invalid", "PWM Rate"=0.0}}}, "PID Ref"=refnum}, "Drivetrain"=w6, "PID Ref"=w1) -> (w11:T22)
  n21 = call "Drive Controller Initialization.vi"("Subsystem Name"=w18, "Default Command"=w14) -> ("Current Command"=w16:T37)  [unwired: 9 in]
  n22 = disable-structure shown="Disabled" {
    disable-tunnel: w13 -> [w37 _]
    frame Disabled {
      n23 = while {
        tunnel: w37 -> [w39]
        stop <- FALSE stop-if-true
        n24 = call "Drive Controller Interactive Check.vi"("Interactive Command In"="Interactive Values", "Default Command"=w39, "Buttons"="Buttons") -> ("Interactive Command Out"=w41:T7, "Trace String"=w42:string, "Schedule"=w43:bool)  [unwired: 6 in]
        n25 = case shown="False" w43 {
          tunnel: [w52 w60] -> w44
          tunnel: [w51 w56] -> w45
          tunnel: w42 -> [_ w58]
          tunnel: w41 -> [_ w57]
          frame False {
            n26 = Tick Count (ms)() -> (millisecond timer value=w55:u32)
            n27 = call "Read Drive Operation.vi"() -> ("Command Info"=w49:T35, "SubSystem Data"=w48:T7)  [unwired: 9 in, 1 out]
            n28 = Unbundle(w48) -> ("Operation"=w53:T8, "Left Setpoint"=w50:dbl)  [unwired: 3 out]
            n29 = Unbundle(w49) -> ("Status"=w52:T9)  [unwired: 2 out]
            n30 = Subtract(x=w55, y=w53) -> (x-y=w54:u32)
            n31 = Bundle(w54, "Left Setpoint"=w50) -> (w51:cluster{u32, "Left Setpoint":dbl})  [unwired: 1 in]
          }
          frame True {
            n32 = call "Drive Command Helper.vi"("Description"=w58, "SubSystem Data"=w57) -> ("Command Info Out"=w59:T35, "Command Timing"=w56:cluster{"Start Time (ms)":u32, "Iterations":i32})  [unwired: 7 in, 1 out]
            n33 = Unbundle(w59) -> ("Status"=w60:T9)  [unwired: 2 out]
          }
        }
        "Status" <- w44
        "Command Timing" <- w45
        n34 = Wait (ms)(milliseconds to wait=u32 20) -> ()  [unwired: 1 out]
      }
    }
    frame Enabled {
    }
  }
  n35 = vi-ref "Reserve Drive.vi"() -> (w15:refnum<vi>)
  n36 = while {
    shift-right: [w68] -> _
    shift-left: w16 -> [w74]
    tunnel: [w63] -> _
    tunnel: "error in" -> [_]
    tunnel: w15 -> [_]
    shift-right: [w61] -> _
    shift-left: w11 -> [w61]
    tunnel: w7 -> [_]
    i -> [w63]
    stop <- FALSE stop-if-true
    # "Current Command"
    # "Drive Controller Loop"
    n37 = Unbundle(w74) -> ("SubSystem Data"=w87:T7, w76:cluster{"Start Time (ms)":u32, "Iterations":i32})  [unwired: 1 out]
    n38 = Unbundle By Name(w87) -> ("Operation"=w86:T8, "Left Setpoint"=w85:dbl, "Right Setpoint"=w84:dbl, "Duration"=w83:dbl, "Data"=w69:variant)
    n39 = Tick Count (ms)() -> (millisecond timer value=w82:u32)
    n40 = disable-structure shown="Enabled" {
      disable-tunnel: w63 -> [w92 _]
      disable-tunnel: [w91 _] -> w62
      frame Enabled {
        n41 = shared-variable ".\\OdometryData.lvlib\\Odometry"() -> (w97:T41)  [unwired: 1 in, 1 out]
        n42 = Equal To 0?(x=w92) -> (x = 0?=w99:bool)
        n43 = call "DMA Odometry Calculate.vi"("Reset?"=w99, "Encoder Factor"="Encoder Factor") -> ("Sequence Lost"=w94:u16, "Pose"=w98:T11, "Right Encoder Raw"=w89:dbl, "Left Encoder Raw"=w90:dbl)  [unwired: 5 in, 1 out]
        "Pose" <- w98
        n44 = Unbundle By Name(w97) -> ("Late Iterations"=w95:u32)
        n45 = To Unsigned Long Integer(number=w94) -> (unsigned 32bit integer=w93:u32)
        n46 = Add(x=w95, y=w93) -> (x+y=w96:u32)
        n47 = Bundle By Name(cluster=w97, "Pose2d"=w98, "Late Iterations"=w96, "Left Encoder"=w90, "Right Encoder"=w89) -> (w91:T41)
        n48 = shared-variable ".\\OdometryData.lvlib\\Odometry"(w91) -> ()  [unwired: 1 in, 1 out]
      }
      frame Disabled {
      }
    }
    n49 = case shown="\"Drive for Distance\"" w86 {
      tunnel: [w141 w163 20.0 ("Wait ms") 30.0 ("Wait ms") 30.0 ("Wait ms") 50.0 0.0 ("Wait ms") 30.0 ("Wait ms")] -> w75
      tunnel: [w138 w169 FALSE ("ignore previous (F)") w215 w248 FALSE ("ignore previous (F)") TRUE ("ignore previous (F)") w267] -> w80
      tunnel: w76 -> [w137 w171 w180 _ w251 _ _ w274]
      tunnel: [w134 w168 w183 w205 w218 w257 w263 w272] -> w72
      tunnel: [w133 w167 w182 w204 w217 w257 w263 w271] -> w71
      tunnel: w85 -> [w136 w168 w181 w203 _ _ _ w270]
      tunnel: w84 -> [w135 w167 _ _ _ _ _ _]
      tunnel: w83 -> [_ w162 _ _ _ _ _ _]
      tunnel: w82 -> [w130 w166 w178 _ w244 _ _ _]
      tunnel: w62 -> [_ _ _ w196 w237 _ _ w273]
      tunnel: w69 -> [_ _ _ _ w254 _ _ _]
      tunnel: ["Control Mode" _ _ Spark_MAX_Control_Type."Velocity" ("Control Mode") Spark_MAX_Control_Type."Velocity" ("Control Mode") _ Spark_MAX_Control_Type."Percent VBus" ("Control Mode") w268] -> w67
      tunnel: [w128 _ _ _ w241 _ _ w266] -> w66
      tunnel: [w127 _ _ _ w240 _ _ w265] -> w65
      tunnel: "Feed Forward" -> [w131 _ _ _ w238 _ _ w264]
      tunnel: w61 -> [_ _ _ _ _ _ _ w269]
      frame "Immediate", Default {
        w141 = 100.0  # Wait ms
        n50 = Unbundle(w137) -> ("Start Time (ms)"=w129:u32, "Iterations"=w126:i32)
        n51 = Subtract(x=w130, y=w129) -> (x-y=w139:u32)
        n52 = Greater?(x=w139, y=u32 50 ("Left Motor")) -> (0:w138:bool)
        n53 = Equal To 0?(x=w126) -> (x = 0?=w125:bool)
        n54 = case shown="\"Velocity\"" "Control Mode" {
          tunnel: w136 -> [w143 w161]
          tunnel: w135 -> [w142 w160]
          tunnel: [w143 w145] -> w134
          tunnel: [w142 w144] -> w133
          tunnel: w131 -> [_ w154]
          tunnel: w130 -> [_ w153]
          tunnel: w129 -> [_ w152]
          tunnel: [_ w150] -> w128
          tunnel: [_ w149] -> w127
          tunnel: w125 -> [_ w148]
          frame "Percent VBus", Default {
          }
          frame "Velocity" {
            n55 = local read "Max Velocity"() -> (w159:dbl)
            n56 = Subtract(x=w153, y=w152) -> (x-y=w156:u32)
            n57 = shared-variable ".\\OdometryData.lvlib\\Velocity"() -> (w146:T42)  [unwired: 1 in, 1 out]
            n58 = Divide(x=w156, y=1000.0) -> (x/y=w158:dbl)
            n59 = feedback #1() -> (w157:dbl)  [unwired: 1 in]
            n60 = feedback-in #1(w158) -> ()
            n61 = Multiply(x=w161, y=w159) -> (x*y=w145:dbl)
            n62 = Multiply(x=w160, y=w159) -> (x*y=w144:dbl)
            n63 = Subtract(x=w158, y=w157) -> (x-y=w151:dbl)
            n64 = Bundle By Name(cluster=w146, "Left Setpoint"=w145, "Right Setpoint"=w144) -> (w147:T42)
            n65 = call "Simple Motor Feedforward.vi"("Reset? (F)"=w148, "dt"=w151, "Feed Forward Constants"=w154, "Velocity Reference"=w145) -> ("Feedforward"=w150:dbl)  [unwired: 7 in]
            n66 = shared-variable ".\\OdometryData.lvlib\\Velocity"(w147) -> ()  [unwired: 1 in, 1 out]
            n67 = call "Simple Motor Feedforward.vi"("Reset? (F)"=w148, "dt"=w151, "Feed Forward Constants"=w154, "Velocity Reference"=w144) -> ("Feedforward"=w149:dbl)  [unwired: 7 in]
          }
        }
      }
      frame "Drive for Time" {
        n68 = Unbundle(w171) -> ("Start Time (ms)"=w170:u32)  [unwired: 1 out]
        n69 = Subtract(x=w166, y=w170) -> (x-y=w174:u32)
        n70 = Multiply(x=w162, y=1000.0) -> (x*y=w173:dbl)
        n71 = Subtract(x=w173, y=w174) -> (x-y=w165:dbl)
        n72 = Max & Min(x=w165, y=50.0) -> (min(x,y)=w163:dbl)  [unwired: 1 out]
        n73 = Less Or Equal To 0?(x=w165) -> (x <= 0?=w169:bool)
      }
      frame "Drivetrain Char" {
        # "\"Quasi-static ramp can be used to DT break-in"
        n74 = Unbundle By Name(w180) -> ("Start Time (ms)"=w179:u32)
        n75 = Subtract(x=w178, y=w179) -> (x-y=w177:u32)
        n76 = case shown="\"quasi-static ramp\"" "Test" {
          tunnel: [w185 w188 w195] -> w183
          tunnel: [w185 w188 w195] -> w182
          tunnel: w181 -> [_ w190 w195]
          tunnel: w177 -> [_ w194 _]
          frame "", Default {
            w185 = 0.0
          }
          frame "quasi-static ramp" {
            w187 = 10.0  # volts max
            n77 = Divide(x=w190, y=w187) -> (x/y=w191:dbl)
            n78 = Divide(x=w194, y=1000.0 ("amplitude")) -> (x/y=w193:dbl)
            n79 = call <vilib>:"Triangle Wave PtByPt.vi"("time"=w193, "frequency"=w191, "amplitude"=w187) -> ("triangle wave"=w189:dbl)  [unwired: 1 in]
            n80 = Divide(x=w189, y=12.0) -> (x/y=w188:dbl)
          }
          frame "step-voltage acceleration" {
          }
        }
      }
      frame "Pure Pursuit" {
        n81 = Max & Min(x=w203, y="Max Velocity") -> (max(x,y)=w201:dbl)  [unwired: 1 out]
        n82 = call "Pure Pursuit.vi"("Lookahead"="Lookahead", "Trackwidth"="Trackwidth", "kffv"="kffv", "kffa"="kffa", "Odometry"=w196, "Max Velocity"=w201, "Max Accel"="Max Accel") -> ("Left Velocity"=w204:dbl, "Right Velocity"=w205:dbl, "Target Point"=w210:T39, "Close Point"=w209:T39, "Finished?"=w215:bool, "index out"=w198:i32, "Curvature"=w208:dbl)  [unwired: 1 in, 1 out]
        n83 = Bundle(cluster=T38 {"Target Point"={"x"=0.0, "y"=0.0, "heading"=0.0, "curvature"=0.0, "total distance"=0.0, "velocity expected"=0.0}, "Close Point"={"x"=0.0, "y"=0.0, "heading"=0.0, "curvature"=0.0, "total distance"=0.0, "velocity expected"=0.0}, "Curvature"=0.0, "index out"=0} ("Pure Pursuit"), "Target Point"=w210, "Close Point"=w209, "Curvature"=w208, "index out"=w198) -> (w199:T38)
        n84 = shared-variable ".\\Pure Pursuit.lvlib\\Pure Pursuit"(w199) -> ()  [unwired: 1 in, 1 out]
      }
      frame "Ramsete" {
        w216 = 0.03 ("dt")
        n85 = Unbundle By Name(w251) -> ("Start Time (ms)"=w246:u32, "Iterations"=w243:i32)
        n86 = Unbundle By Name(w237) -> ("Pose2d"=w236:T11)
        n87 = Equal To 0?(x=w243) -> (x = 0?=w229:bool)
        n88 = Subtract(x=w244, y=w246) -> (x-y=w250:u32)
        n89 = Get Variant Attribute(Variant=w254, name="ramsete_traj", default value (empty Variant)=T40[] [] ("states")) -> (value=w230:T40[])  [unwired: 1 in, 3 out]
        n90 = Divide(x=w250, y=1000.0) -> (x/y=w226:dbl)
        n91 = Index Array(array=w230) -> (element=w235:T40)  [unwired: 1 in]
        n92 = feedback-in #2(w226) -> ()
        n93 = feedback #2() -> (w239:dbl)  [unwired: 1 in]
        n94 = Unbundle By Name(w235) -> ("pose"=w234:T11)
        n95 = Select(t=w234, s=w229, f=w236) -> (s? t:f=w222:T11)
        n96 = Unbundle By Name(w222) -> ("Rotation2d.Theta"=w221:dbl)
        n97 = call "Ramsete Command.vi"("Trackwidth"="Trackwidth", "Reset? (F)"=w229, "timestamp (s)"=w226, "Trajectory"=w230, "Pose2d"=w222) -> ("Finished?"=w248:bool, "Right Velocity Ref"=w217:dbl, "Left Velocity Ref"=w218:dbl)  [unwired: 4 in]
        n98 = Subtract(x=w226, y=w239) -> ()  [unwired: 1 out]
        n99 = Add(x=w218, y=w217) -> (x+y=w225:dbl)
        n100 = Divide(x=w225, y=2.0) -> (x/y=w223:dbl)
        n101 = Bundle By Name(cluster=T40 {"t"=0.0, "velocity"=0.0, "acceleration"=0.0, "pose"={"Translation2d"={"x"=0.0, "y"=0.0}, "Rotation2d"={"Theta"=0.0}}, "curvature"=0.0} ("State"), "t"=w226, "velocity"=w223, "pose.Rotation2d.Theta"=w221) -> (w227:T40)
        n102 = call <vilib>:"Plot Trajectory PtbyPt.vi"("Reset? (F)"=w229, "State"=w227) -> ("Telemetry"=w231:cluster{dbl[], dbl[]}[])  [unwired: 9 in]
        n103 = shared-variable ".\\OdometryData.lvlib\\Velocity"() -> (w219:T42)  [unwired: 1 in, 1 out]
        n104 = call <vilib>:"Plot Trajectory.vi"("states"=w230) -> ("Telemetry"=w233:cluster{dbl[], dbl[]}[])  [unwired: 9 in, 1 out]
        n105 = case shown="True" w229 {
          selector: w229 -> [_ w255]
          tunnel: w234 -> [_ w256]
          frame False {
          }
          frame True {
            n106 = global write "Odometry Set.vi" "Pose2d"(w256) -> ()
            n107 = global write "Odometry Set.vi" "Set?"(w255) -> ()
          }
        }
        n108 = Build Array (concatenate)(w233, w231) -> (→"Telemetry":cluster{dbl[], dbl[]}[])
        n109 = Bundle By Name(cluster=w219, "Left Setpoint"=w218, "Right Setpoint"=w217) -> (w220:T42)
        n110 = shared-variable ".\\OdometryData.lvlib\\Velocity"(w220) -> ()  [unwired: 1 in, 1 out]
        n111 = call "Simple Motor Feedforward.vi"("Reset? (F)"=w229, "dt"=w216, "Feed Forward Constants"=w238, "Velocity Reference"=w218) -> ("Feedforward"=w241:dbl)  [unwired: 7 in]
        n112 = call "Simple Motor Feedforward.vi"("Reset? (F)"=w229, "dt"=w216, "Feed Forward Constants"=w238, "Velocity Reference"=w217) -> ("Feedforward"=w240:dbl)  [unwired: 7 in]
      }
      frame "Reserve" {
        w257 = 0.0  # Don't move motors while reserved
      }
      frame "Turn to Angle" {
        w263 = 0.0 ("Don't move motors while reserved")
      }
      frame "Drive for Distance" {
        n113 = disable-structure shown="Enabled" {
          disable-tunnel: w274 -> [w282 w301]
          disable-tunnel: w273 -> [w281 w298]
          disable-tunnel: [w280 w285] -> w272
          disable-tunnel: [w279 w284] -> w271
          disable-tunnel: w270 -> [w278 w296]
          disable-tunnel: w269 -> [_ w300]
          disable-tunnel: [_ Spark_MAX_Control_Type."Velocity" ("Control Mode")] -> w268
          disable-tunnel: [_ w294] -> w267
          disable-tunnel: [_ w293] -> w266
          disable-tunnel: [_ w292] -> w265
          disable-tunnel: w264 -> [_ w291]
          frame Disabled {
            n114 = Unbundle By Name(w282) -> ("Iterations"=w276:i32)  [unwired: 1 out]
            n115 = call "Drive Straight PID.vi"("Iteration"=w276, "target distance"=w278, "Period (ms)"=i64 30, "Odometry"=w281) -> ("Right Axis"=w279:dbl, "Left Axis"=w280:dbl)  [unwired: 6 in]
          }
          frame Enabled {
            w288 = 0.03 ("dt (s)")
            n116 = Unbundle(w301) -> ("Iterations"=w290:i32)  [unwired: 1 out]
            n117 = Unbundle By Name(w300) -> ("PID Ref"=w299:refnum<data-value>)
            n118 = call "Drive Straight Profiled PID.vi"("Gyro PIDF"="Gyro PIDF", "Iteration"=w290, "Position Tolerance"="Drive Distance Tolerance", "dt (s)"=w288, "target distance"=w296, "Odometry"=w298, "PID Ref in"=w299) -> ("At Target?"=w294:bool, "Right Speed"=w284:dbl, "Left Speed"=w285:dbl)  [unwired: 2 in]
            n119 = shared-variable ".\\OdometryData.lvlib\\Velocity"() -> (w286:T42)  [unwired: 1 in, 1 out]
            n120 = Equal To 0?(x=w290) -> (x = 0?=w289:bool)
            n121 = Bundle By Name(cluster=w286, "Left Setpoint"=w285, "Right Setpoint"=w284) -> (w287:T42)
            n122 = call "Simple Motor Feedforward.vi"("Reset? (F)"=w289, "dt"=w288, "Feed Forward Constants"=w291, "Velocity Reference"=w285) -> ("Feedforward"=w293:dbl)  [unwired: 7 in]
            n123 = call "Simple Motor Feedforward.vi"("Reset? (F)"=w289, "dt"=w288, "Feed Forward Constants"=w291, "Velocity Reference"=w284) -> ("Feedforward"=w292:dbl)  [unwired: 7 in]
            n124 = shared-variable ".\\OdometryData.lvlib\\Velocity"(w287) -> ()  [unwired: 1 in, 1 out]
          }
        }
      }
    }
    n125 = Unbundle By Name(w74) -> ("SubSystem Data.Operation"=w73:T8)
    n126 = call "Drive Check for New Command.vi"("input cluster"=w74, "Wait time (ms)"=w75, "Finished?"=w80) -> ("Completion"=w81:T9, "Subsystem Name"=w77:string, "Current Command"=w78:T7, "Initial Trace String"=w79:string, "Next Command"=w68:T43)  [unwired: 4 in]
    n127 = case shown="\"Successful\", \"Aborted\"" w81 {
      selector: w81 -> [_ w102]
      tunnel: w79 -> [_ w106]
      tunnel: w78 -> [_ w107]
      tunnel: w77 -> [_ w104]
      tunnel: w73 -> [_ w103]
      tunnel: w68 -> [_ w101]
      frame "Incomplete", Default {
        # "Continuing current command"
      }
      frame "Successful", "Aborted" {
        # "Report and setup for next command"
        n128 = case shown="\"Pure Pursuit\", \"Ramsete\"" w103 {
          tunnel: w107 -> [w111 _ _]
          tunnel: w106 -> [w110 w115 w121]
          tunnel: [w109 w115 w121] -> w105
          tunnel: w102 -> [_ _ w120]
          tunnel: w101 -> [_ _ w117]
          frame "Reserve", Default {
            n129 = Unbundle By Name(w111) -> ("Left Setpoint"=w113:dbl, "Right Setpoint"=w114:dbl, "Duration"=w108:dbl)
            n130 = Format Into String(format string="L %.1f, R %.1f, D %f", initial string=w110, w113, w114, w108) -> (resulting string=w109:string)  [unwired: 1 in, 1 out]
          }
          frame "Read Current" {
            # "Placeholder for \ncomplex commands\nwith cleanup"
          }
          frame "Pure Pursuit", "Ramsete" {
            n131 = Unbundle By Name(w117) -> ("SubSystem Data.Operation"=w116:T8)
            n132 = Equal?(x=Completion_Status."Aborted", y=w120) -> (x = y?=w118:bool)
            n133 = case shown="True" w118 {
              tunnel: w116 -> [_ w122]
              frame False {
              }
              frame True {
                n134 = Format Into String(format string="Aborted Path Followeing for: %s", w122) -> (resulting string=w124:string)  [unwired: 2 in, 1 out]
                n135 = call <vilib>:"WPI_UtilitiesFRC SendMessageToConsole.vi"("Message"=w124) -> ()  [unwired: 14 in, 1 out]
              }
            }
          }
        }
        "Current\nCmd" <- w105
        n136 = call <vilib>:"Trace Results.vi"("Status of previous command"=w102, "Description"=w105, "Subsystem"=w104) -> ()  [unwired: 9 in]
      }
    }
    n137 = Unbundle By Name(w61) -> ("Drivetrain"=w70:T17)
    n138 = call "CAN 6 SPARK MAX Motor Set Value.vi"("Right Feed Forward (volts)"=w65, "Left Feed Forward (volts)"=w66, "Control Mode"=w67, "Right Power"=w71, "Left Power"=w72, "Drivetrain"=w70) -> ()  [unwired: 6 in]
  }
  n139 = while {
    tunnel: w9 -> [w313]
    tunnel: w8 -> [w310]
    tunnel: w1 -> [w304]
    stop <- FALSE stop-if-true
    # "Tunable PIDF!"
    n140 = feedback #3(T10 {"P Gain"=0.0, "I Gain"=0.0, "D Gain"=0.0, "F Gain"=0.0, "I Zone"=0.0, "Min Output"=0.0, "Max Output"=0.0} ("PID Constants")) -> (w319:T10)
    n141 = Not Equal?(x="PID Constants Drivetrain", y=w319) -> (x != y?=w314:T44)
    n142 = Cluster To Array(cluster=w314) -> (array=w315:bool[])
    n143 = Or Array Elements(Boolean array=w315) -> (logical OR=w317:bool)
    n144 = First Call?() -> (First Call?: T/F=w307:bool)
    n145 = Or(x=w307, y=w317) -> (x .or. y?=w308:bool)
    n146 = Wait (ms)(milliseconds to wait=u32 200) -> ()  [unwired: 1 out]
    n147 = case shown="True" w308 {
      tunnel: w313 -> [_ w323]
      tunnel: "PID Constants Drivetrain" -> [_ w322]
      tunnel: [w320 w322] -> w318
      tunnel: w319 -> [w320 _]
      tunnel: w310 -> [_ w321]
      frame False {
      }
      frame True {
        n148 = call <vilib>:"Spark MAX Set PIDF Constants.vi"("PID Constants"=w322, "MotorControlDeviceRef"=w323) -> ()  [unwired: 8 in, 2 out]
        n149 = call <vilib>:"Spark MAX Set PIDF Constants.vi"("PID Constants"=w322, "MotorControlDeviceRef"=w321) -> ()  [unwired: 8 in, 2 out]
      }
    }
    n150 = feedback-in #3(w318) -> ()
    n151 = call <vilib>:"PID Set Contraints.vi"("Profiled Contraints"="Profiled Contraints", "Output Range"="Output Range", "PID Ref"=w304) -> ("PID Ref"=w306:refnum<data-value>)  [unwired: 8 in]
    n152 = call <vilib>:"PID Set Gains.vi"("PIDF Gains"="PIDF Gains", "PID Ref"=w306) -> ()  [unwired: 9 in, 1 out]
  }
